vi "vipm_ApplyVIPCFile.vi"(8 "error in (no error)":errorcluster, 11 "CommandLine":string[](array[string])=["<lvAPT_Sync>\\lvapt_devlopment_palette"]) -> (0 "error out":errorcluster, 2 "test details":string)   [LabVIEW 2019]
uses:
  <vilib>/JKI/VIPM API/VIPM API_vipm_api.lvlib
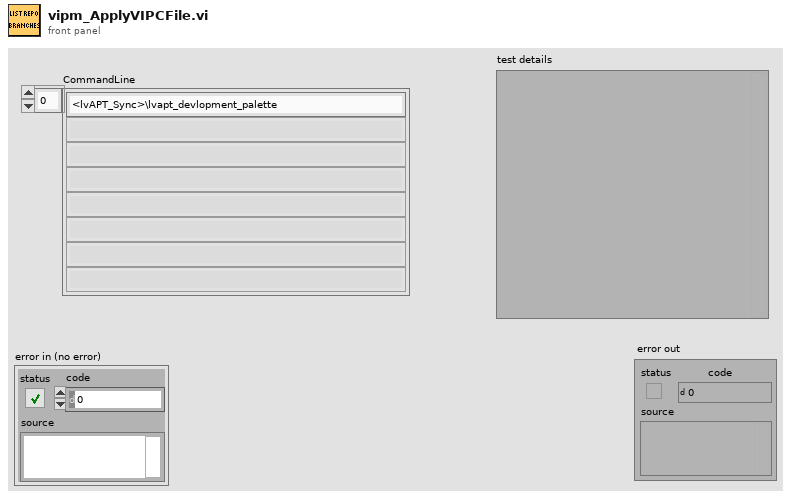
[diagram p1: front panel]
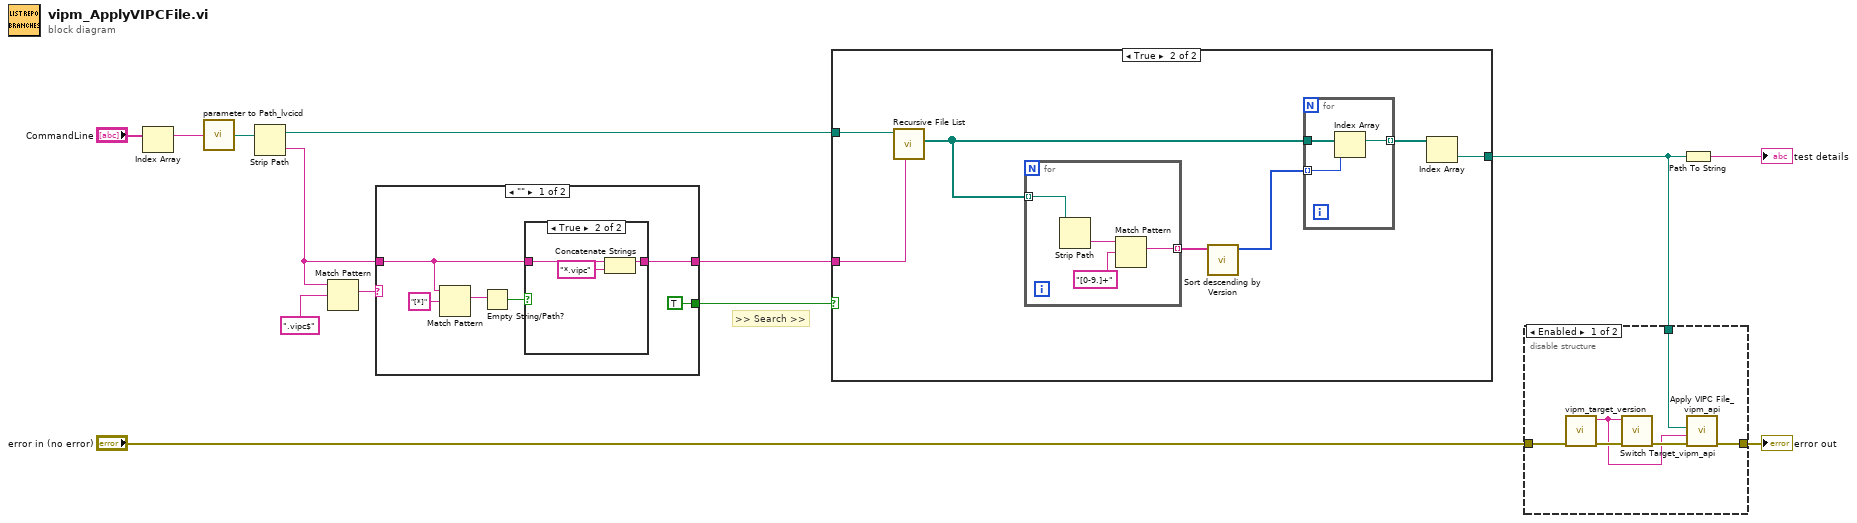
[diagram p0: block diagram]
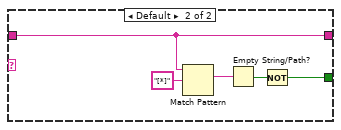
[diagram p5: hidden frame]
diagram:
  # ">> Search >>"
  n1 = Index Array(array="CommandLine") -> (element=w9:string)  [unwired: 1 in]
  n2 = call "parameter to Path_lvcicd.vi"("String"=w9) -> ("Path"=w8:path)
  n3 = Strip Path(path=w8) -> (stripped path=w7:path, name=w4:string)
  n4 = Match Pattern(string=w4, regular expression=".vipc$") -> (match substring=w5:string)  [unwired: 1 in, 3 out]
  n5 = case shown="\"\"" w5 {
    tunnel: w4 -> [w14 w28]
    tunnel: [w15 w28] -> w3
    tunnel: [TRUE w24] -> w2
    frame "" {
      n6 = Match Pattern(string=w14, regular expression="[*]") -> (match substring=w18:string)  [unwired: 1 in, 3 out]
      n7 = Empty String/Path?(string/path=w18) -> (empty?=w17:bool)
      n8 = case shown="True" w17 {
        tunnel: [w20 w22] -> w15
        tunnel: w14 -> [w20 w23]
        frame False {
        }
        frame True {
          n9 = Concatenate Strings(w23, "*.vipc" ("string")) -> (w22:string)
        }
      }
    }
    frame Default {
      n10 = Match Pattern(string=w28, regular expression="[*]") -> (match substring=w26:string)  [unwired: 1 in, 3 out]
      n11 = Empty String/Path?(string/path=w26) -> (empty?=w25:bool)
      n12 = Not(x=w25) -> (.not. x?=w24:bool)
    }
  }
  n13 = case shown="True" w2 {
    tunnel: w7 -> [w29 w36]
    tunnel: [w29 w35] -> w11
    tunnel: w3 -> [_ w32]
    frame False {
    }
    frame True {
      n14 = call <vilib>:"Recursive File List.vi"("pattern"=w32, "Folder Path"=w36) -> ("All Files in Dir"=w31:path[])  [unwired: 5 in, 4 out]
      n15 = for {
        tunnel: w31 -> [w38] mode=indexing
        tunnel: [w37] -> w30 mode=indexing
        n16 = Strip Path(path=w38) -> (name=w39:string)  [unwired: 1 out]
        n17 = Match Pattern(string=w39, regular expression="[0-9.]+") -> (match substring=w37:string)  [unwired: 1 in, 3 out]
      }
      n18 = call "Sort descending by Version.vi"("Array"=w30) -> ("Sorted Pointers"=w34:i32[])  [unwired: 10 in]
      n19 = for {
        tunnel: w31 -> [w43]
        tunnel: [w42] -> w33 mode=indexing
        tunnel: w34 -> [w41] mode=indexing
        n20 = Index Array(array=w43, index=w41) -> (element=w42:path)
      }
      n21 = Index Array(array=w33) -> (element=w35:path)  [unwired: 1 in]
    }
  }
  n22 = disable-structure shown="Enabled" {
    disable-tunnel: [w48 _] -> w13
    disable-tunnel: w11 -> [w47 _]
    disable-tunnel: "error in (no error)" -> [w46 _]
    frame Enabled {
      n23 = call "vipm_target_version.vi"() -> ("vipm Taget version"=w44:string)  [unwired: 11 in]
      n24 = call <vilib>:"Switch Target_vipm_api.vi"("error in (no error)"=w46, "LabVIEW Version"=w44) -> ("error out"=w45:errorcluster)  [unwired: 9 in]
      n25 = call <vilib>:"Apply VIPC File_vipm_api.vi"("error in (no error)"=w45, "LabVIEW Version"=w44, "VIPC File"=w47) -> ("error out"=w48:errorcluster)  [unwired: 8 in]
    }
    frame Disabled {
    }
  }
  "error out" <- w13
  n26 = Path To String(path=w11) -> (string=→"test details":string)
